vi "FindHorizontalEdges.vi"(8 "error in (no error)":errorcluster, 10 "Coordinate System":T2 {"Measurement System"."Axis Reference" items=["Direct", "Indirect"]; "Measurement System"."Angle (deg)" format="%.2f"; "Measurement System"."Origin"."Y" format="%.2f"; "Measurement System"."Origin"."X" format="%.2f"; "Reference System"."Axis Reference" items=["Direct", "Indirect"]; "Reference System"."Angle (deg)" format="%.2f"; "Reference System"."Origin"."Y" format="%.2f"; "Reference System"."Origin"."X" format="%.2f"}, 11 "Image":T1) -> (0 "error out":errorcluster, 2 "Straight Edges":T3(array[cluster]) {"Point2 (Real-World)"."Y" format="%.2f"; "Point2 (Real-World)"."X" format="%.2f"; "Point1 (Real-World)"."Y" format="%.2f"; "Point1 (Real-World)"."X" format="%.2f"; "Point2 (Pixels)"."Y" format="%.2f"; "Point2 (Pixels)"."X" format="%.2f"; "Point1 (Pixels)"."Y" format="%.2f"; "Point1 (Pixels)"."X" format="%.2f"}, 3 "Image 2":T1(plugin-control))   [LabVIEW 2017]
uses:
  <vilib>/vision/Image Controls.llb/IMAQ Image.ctl
  <vilib>/vision/Measure.llb/Edge Options.ctl
  <vilib>/vision/Measure.llb/Edge Polarity.ctl
  <vilib>/vision/Measure.llb/Straight Edge Options.ctl
  <vilib>/vision/Measure.llb/Straight Edge Process.ctl
  <vilib>/vision/NI_Vision_Development_Module.lvlib
panel:
  out "Image 3":T1(plugin-control)
  out "Coordinate System (duplicate)":T2 {"Measurement System"."Axis Reference" items=["Direct", "Indirect"]; "Measurement System"."Angle (deg)" format="%.2f"; "Measurement System"."Origin"."Y" format="%.2f"; "Measurement System"."Origin"."X" format="%.2f"; "Reference System"."Axis Reference" items=["Direct", "Indirect"]; "Reference System"."Angle (deg)" format="%.2f"; "Reference System"."Origin"."Y" format="%.2f"; "Reference System"."Origin"."X" format="%.2f"}
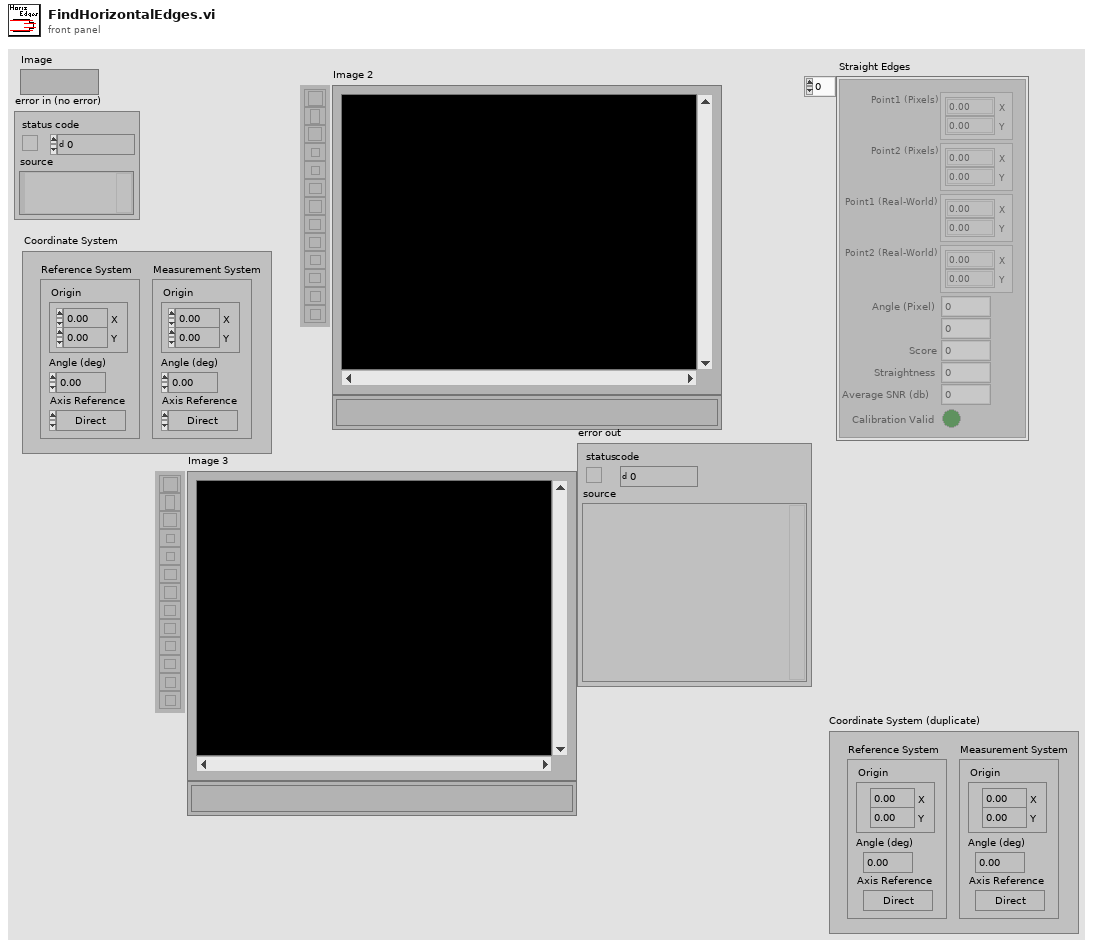
[diagram p1: front panel]
types:
  T1 = typedef "IMAQ Image.ctl" = refnum<image>
  T2 = typedef "IMAQ Coordinate System" = cluster{"Reference System":cluster{"Origin":cluster{"X":sgl, "Y":sgl}, "Angle (deg)":sgl, "Axis Reference":u32}, "Measurement System":cluster{"Origin":cluster{"X":sgl, "Y":sgl}, "Angle (deg)":sgl, "Axis Reference":u32}}
  T3 = cluster{"Point1 (Pixels)":cluster{"X":sgl, "Y":sgl}, "Point2 (Pixels)":cluster{"X":sgl, "Y":sgl}, "Point1 (Real-World)":cluster{"X":sgl, "Y":sgl}, "Point2 (Real-World)":cluster{"X":sgl, "Y":sgl}, "Angle (Pixel)":dbl, "Angle (Real-World)":dbl, "Score":dbl, "Straightness":dbl, "Average SNR (db)":dbl, "Calibration Valid":bool}[]
  T4 = typedef "Straight Edge Options.ctl" = cluster{"Number of Lines":i32, "Type":T5, "Min. Score":dbl, "Max. Score":dbl, "Orientation":dbl, "Angle Range":dbl, "Angle Tolerance":dbl, "Step Size":u32, "Min. SNR (db)":dbl, "Min. Points (%)":dbl, "Hough Iterations":i32}
  T5 = typedef "Straight Edge Process.ctl" = enum32{"First Edge Rake", "Best Edge Rake", "Hough Edge Rake", "First Edge Projection", "Best Edge Projection"}
  T6 = typedef "Edge Options.ctl" = cluster{"Edge Polarity":T7, "Kernel Size":u32, "Width":u32, "Minimum Edge Strength":sgl, "Interpolation Type":enum32{"Zero Order", "Bilinear", "Quadratic", "Cubic", "Bilinear Fixed"}, "Data Processing Method":enum32{"Average", "Median"}}
  T7 = typedef "Edge Polarity.ctl" = u32
  T8 = cluster{"Search Direction":u32, "Edge Options":T6, "Show Search Area":bool, "Show Search Lines":bool, "Show Edges Found":bool, "Show Result":bool, "Search Area Color":u32, "Search Lines Color":u32, "Edge Locations Color":u32, "Result Color":u32, "Overlay Group Name":string}
  T9 = typedef "IMAQ Rectangle" = cluster{"Left":i32, "Top":i32, "Right":i32, "Bottom":i32, "Rotation":dbl}
  T10 = typedef "ROI Descriptor" = cluster{"Global Rectangle":i32[], "Contours":cluster{"ID":enum32{"External", "Internal"}, "Type":u32, "Coordinates":i32[]}[]}
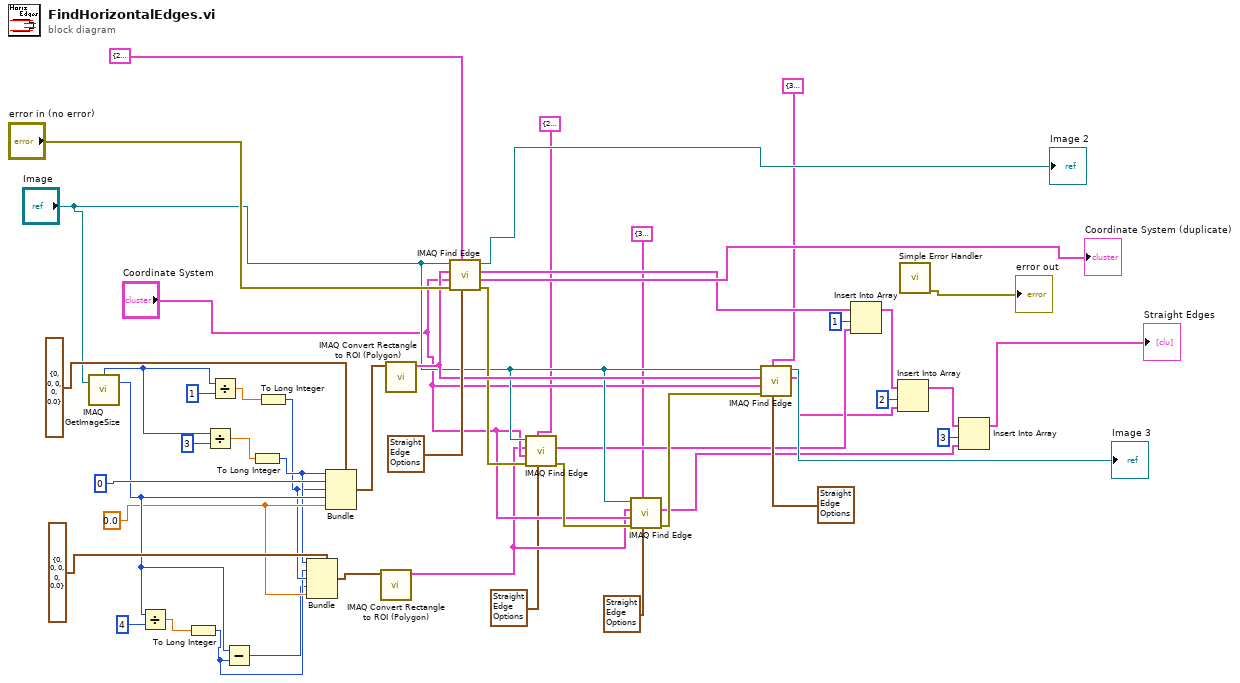
[diagram p0: block diagram]
diagram:
  w14 = 0.0
  n1 = call "IMAQ GetImageSize"("Image"="Image") -> ("Y Resolution"=w15:i32, "X Resolution"=w41:i32)  [unwired: 3 in, 1 out]
  n2 = Divide(x=w15, y=4) -> (x/y=w16:dbl)
  n3 = To Long Integer(number=w16) -> (32bit integer=w11:i32)
  n4 = Divide(x=w41, y=3) -> (x/y=w19:dbl)
  n5 = Divide(x=w41, y=1) -> (x/y=w18:dbl)
  n6 = Subtract(x=w15, y=w11) -> (x-y=w10:i32)
  n7 = To Long Integer(number=w19) -> (32bit integer=w13:i32)
  n8 = To Long Integer(number=w18) -> (32bit integer=w12:i32)
  n9 = Bundle(cluster=T9 {"Left"=0, "Top"=0, "Right"=0, "Bottom"=0, "Rotation"=0.0} ("Rectangle"), "Left"=w13, "Top"=w11, "Right"=w12, "Bottom"=w10, "Rotation"=w14) -> (w9:T9)
  n10 = Bundle(cluster=T9 {"Left"=0, "Top"=0, "Right"=0, "Bottom"=0, "Rotation"=0.0} ("Rectangle"), "Left"=w13, "Top"=0, "Right"=w12, "Bottom"=w15, "Rotation"=w14) -> (w45:T9)
  n11 = call "IMAQ Convert Rectangle to ROI (Polygon)"("Rectangle"=w9) -> ("ROI Descriptor"=w8:T10)  [unwired: 7 in, 2 out]
  n12 = call "IMAQ Convert Rectangle to ROI (Polygon)"("Rectangle"=w45) -> ("ROI Descriptor"=w34:T10)  [unwired: 7 in, 2 out]
  n13 = call "IMAQ Find Edge"("Line Fit Options"=T4 {"Number of Lines"=1, "Type"=enum."First Edge Projection", "Min. Score"=10.0, "Max. Score"=1000.0, "Orientation"=0.0, "Angle Range"=2.0, "Angle Tolerance"=1.0, "Step Size"=7, "Min. SNR (db)"=0.0, "Min. Points (%)"=25.0, "Hough Iterations"=5}, "Options"=T8 {"Search Direction"=2, "Edge Options"={"Edge Polarity"=2, "Kernel Size"=3, "Width"=3, "Minimum Edge Strength"=40.0, "Interpolation Type"=enum."Bilinear Fixed", "Data Processing Method"=enum."Average"}, "Show Search Area"=FALSE, "Show Search Lines"=FALSE, "Show Edges Found"=FALSE, "Show Result"=TRUE, "Search Area Color"=65280, "Search Lines Color"=255, "Edge Locations Color"=16776960, "Result Color"=16711680, "Overlay Group Name"=""}, "error in (no error)"="error in (no error)", "Coordinate System"="Coordinate System", "ROI Descriptor"=w34, "Image"="Image") -> ("error out"=w30:errorcluster, "Coordinate System (duplicate)"=→"Coordinate System (duplicate)":T2, "Straight Edges"=w36:T3, "Image Out"=→"Image 2":T1)  [unwired: 2 in]
  n14 = call "IMAQ Find Edge"("Line Fit Options"=T4 {"Number of Lines"=1, "Type"=enum."First Edge Projection", "Min. Score"=10.0, "Max. Score"=1000.0, "Orientation"=0.0, "Angle Range"=2.0, "Angle Tolerance"=1.0, "Step Size"=7, "Min. SNR (db)"=0.0, "Min. Points (%)"=25.0, "Hough Iterations"=5}, "Options"=T8 {"Search Direction"=2, "Edge Options"={"Edge Polarity"=2, "Kernel Size"=3, "Width"=3, "Minimum Edge Strength"=30.0, "Interpolation Type"=enum."Bilinear Fixed", "Data Processing Method"=enum."Average"}, "Show Search Area"=FALSE, "Show Search Lines"=FALSE, "Show Edges Found"=FALSE, "Show Result"=TRUE, "Search Area Color"=65280, "Search Lines Color"=255, "Edge Locations Color"=16776960, "Result Color"=16711680, "Overlay Group Name"=""}, "error in (no error)"=w30, "Coordinate System"="Coordinate System", "ROI Descriptor"=w8, "Image"="Image") -> ("error out"=w29:errorcluster, "Straight Edges"=w5:T3)  [unwired: 2 in, 2 out]
  n15 = call "IMAQ Find Edge"("Line Fit Options"=T4 {"Number of Lines"=1, "Type"=enum."First Edge Projection", "Min. Score"=10.0, "Max. Score"=1000.0, "Orientation"=0.0, "Angle Range"=2.0, "Angle Tolerance"=1.0, "Step Size"=7, "Min. SNR (db)"=0.0, "Min. Points (%)"=25.0, "Hough Iterations"=5}, "Options"=T8 {"Search Direction"=3, "Edge Options"={"Edge Polarity"=2, "Kernel Size"=3, "Width"=3, "Minimum Edge Strength"=30.0, "Interpolation Type"=enum."Bilinear Fixed", "Data Processing Method"=enum."Average"}, "Show Search Area"=FALSE, "Show Search Lines"=FALSE, "Show Edges Found"=FALSE, "Show Result"=TRUE, "Search Area Color"=65280, "Search Lines Color"=255, "Edge Locations Color"=16776960, "Result Color"=16711680, "Overlay Group Name"=""}, "error in (no error)"=w29, "Coordinate System"="Coordinate System", "ROI Descriptor"=w8, "Image"="Image") -> ("error out"=w28:errorcluster, "Straight Edges"=w3:T3)  [unwired: 2 in, 2 out]
  n16 = call "IMAQ Find Edge"("Line Fit Options"=T4 {"Number of Lines"=1, "Type"=enum."First Edge Projection", "Min. Score"=10.0, "Max. Score"=1000.0, "Orientation"=0.0, "Angle Range"=2.0, "Angle Tolerance"=1.0, "Step Size"=7, "Min. SNR (db)"=0.0, "Min. Points (%)"=25.0, "Hough Iterations"=5}, "Options"=T8 {"Search Direction"=3, "Edge Options"={"Edge Polarity"=2, "Kernel Size"=3, "Width"=3, "Minimum Edge Strength"=30.0, "Interpolation Type"=enum."Bilinear Fixed", "Data Processing Method"=enum."Average"}, "Show Search Area"=FALSE, "Show Search Lines"=FALSE, "Show Edges Found"=FALSE, "Show Result"=TRUE, "Search Area Color"=65280, "Search Lines Color"=255, "Edge Locations Color"=16776960, "Result Color"=16711680, "Overlay Group Name"=""}, "error in (no error)"=w28, "Coordinate System"="Coordinate System", "ROI Descriptor"=w34, "Image"="Image") -> ("Straight Edges"=w4:T3, "Image Out"=→"Image 3":T1)  [unwired: 2 in, 2 out]
  n17 = Insert Into Array(array=w36, index=1, new element=w5) -> (w25:T3)
  n18 = Insert Into Array(array=w25, index=2, new element=w4) -> (w24:T3)
  n19 = call <vilib>:"Simple Error Handler.vi"() -> ("error out"=→"error out":errorcluster)  [unwired: 5 in, 4 out]
  n20 = Insert Into Array(array=w24, index=3, new element=w3) -> (→"Straight Edges":T3)
